vi "Big_array_Rebuild.vi"(10 "숫자형":i32, 11 "Init input":string[](array[string])) -> (3 "추가된 배열":string[][](array[string]))   [LabVIEW 2015]
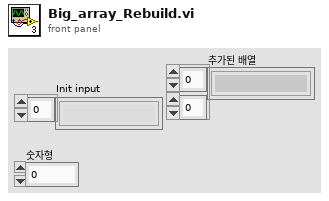
[diagram p1: front panel]
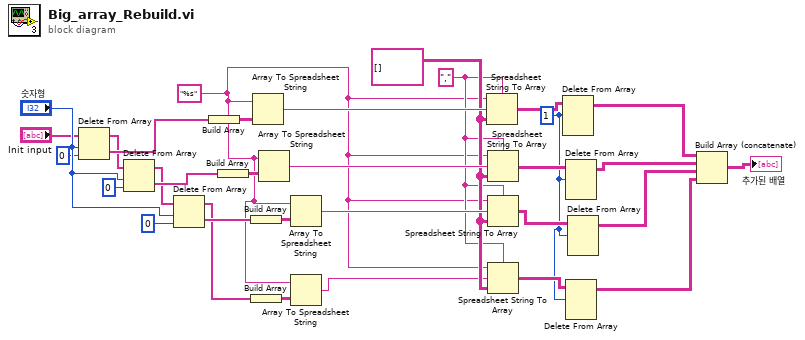
[diagram p0: block diagram]
diagram:
  w1 = 1 ("길이")
  w14 = "," ("구분 문자(탭)")
  w15 = string[][] []
  w10 = "%s" ("포맷 문자열")
  n1 = Delete From Array(array="Init input", length="숫자형", index=0 ("인덱스")) -> (deleted portion=w24:string[], array with subset deleted=w22:string[])
  n2 = Delete From Array(array=w22, length="숫자형", index=0 ("인덱스")) -> (deleted portion=w25:string[], array with subset deleted=w21:string[])
  n3 = Delete From Array(array=w21, length="숫자형", index=0 ("인덱스")) -> (deleted portion=w28:string[], array with subset deleted=w12:string[])
  n4 = Build Array(w24) -> (w23:string[][])
  n5 = Build Array(w25) -> (w26:string[][])
  n6 = Build Array(w28) -> (w27:string[][])
  n7 = Build Array(w12) -> (w13:string[][])
  n8 = Array To Spreadsheet String(array=w23, 3:w10) -> (spreadsheet string=w30:string)  [unwired: 1 in]
  n9 = Array To Spreadsheet String(array=w26, 3:w10) -> (spreadsheet string=w31:string)  [unwired: 1 in]
  n10 = Array To Spreadsheet String(array=w27, 3:w10) -> (spreadsheet string=w32:string)  [unwired: 1 in]
  n11 = Array To Spreadsheet String(array=w13, 3:w10) -> (spreadsheet string=w11:string)  [unwired: 1 in]
  n12 = Spreadsheet String To Array(delimiter (Tab)=w14, format string=w10, spreadsheet string=w30, array type (2D Dbl)=w15) -> (array=w9:string[][])
  n13 = Spreadsheet String To Array(delimiter (Tab)=w14, format string=w10, spreadsheet string=w31, array type (2D Dbl)=w15) -> (array=w7:string[][])
  n14 = Spreadsheet String To Array(delimiter (Tab)=w14, format string=w10, spreadsheet string=w32, array type (2D Dbl)=w15) -> (array=w6:string[][])
  n15 = Spreadsheet String To Array(delimiter (Tab)=w14, format string=w10, spreadsheet string=w11, array type (2D Dbl)=w15) -> (array=w5:string[][])
  n16 = Delete From Array(array=w9, length=w1) -> (array with subset deleted=w8:string[][])  [unwired: 2 in, 1 out]
  n17 = Delete From Array(array=w7, length=w1) -> (array with subset deleted=w4:string[][])  [unwired: 2 in, 1 out]
  n18 = Delete From Array(array=w5, length=w1) -> (array with subset deleted=w2:string[][])  [unwired: 2 in, 1 out]
  n19 = Delete From Array(array=w6, length=w1) -> (array with subset deleted=w3:string[][])  [unwired: 2 in, 1 out]
  n20 = Build Array (concatenate)(w8, w4, w3, w2) -> (→"추가된 배열":string[][])
